vi "Alarm Names.vi"(11 "Alarm":T1 {"value" format="%.2f"; "setpoint" format="%.2f"; "clear time" format="%<%X\n%x>T"; "ack time" format="%<%X\n%x>T"; "set time" format="%<%X\n%x>T"}) -> (1 "Alarm Name":string, 2 "Base Tag Name":string, 3 "Full Variable Name":string)   [LabVIEW 2018, in "Dynamic Shared Variables.lvlib"]
doc: "From the Alarm cluster, determine base tag name and alarm names."
uses:
  Dynamic Shared Variables.lvlib
  <vilib>/regexp/Match Regular Expression.xnode
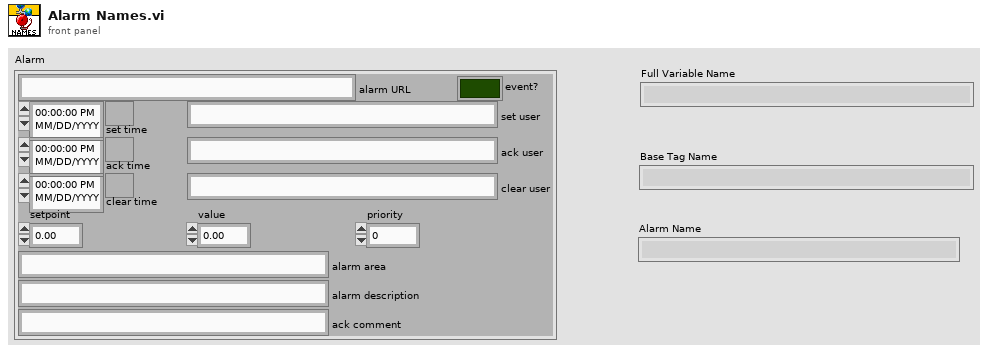
[diagram p1: front panel]
types:
  T1 = cluster{"alarm URL":string, "set time":timestamp, "set user":string, "ack time":timestamp, "ack user":string, "clear time":timestamp, "clear user":string, "setpoint":dbl, "value":dbl, "priority":u32, "alarm area":string, "alarm description":string, "ack comment":string, "event?":bool, "Refnum":u64}
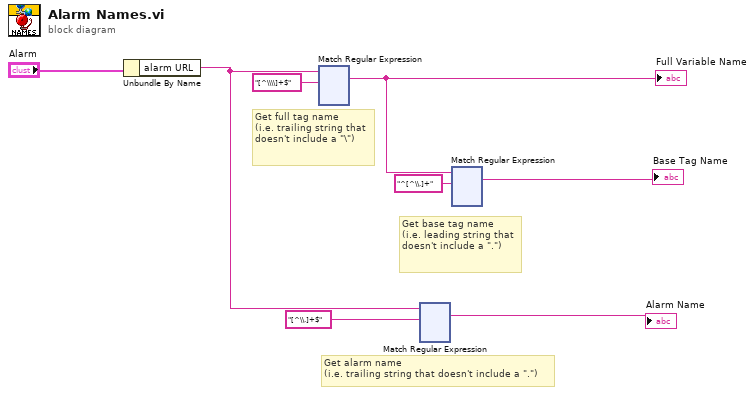
[diagram p0: block diagram]
diagram:
  # "Get base tag name\n(i.e. leading string that doesn't include a \".\")"
  # "Get alarm name\n(i.e. trailing string that doesn't include a \".\")"
  # "Get full tag name\n(i.e. trailing string that doesn't include a \"\\\")"
  n1 = Unbundle By Name("Alarm") -> ("alarm URL"=w4:string)
  n2 = xnode "Match Regular Expression"("input string"=w4, "regular expression"="[^\\\\]+$") -> ("whole match"=w7:string)  [unwired: 4 in, 4 out]
  "Full Variable Name" <- w7
  n3 = xnode "Match Regular Expression"("input string"=w4, "regular expression"="[^\\.]+$") -> ("whole match"=→"Alarm Name":string)  [unwired: 4 in, 4 out]
  n4 = xnode "Match Regular Expression"("input string"=w7, "regular expression"="^[^\\.]+") -> ("whole match"=→"Base Tag Name":string)  [unwired: 4 in, 4 out]
